vi "Property Read.vi"(4 "error in (no error)":errorcluster, 6 "Container State":T2, 7 "Display State In":T1={"Update"=FALSE, "Show advanced"=FALSE, "Fs (Hz)"=100000.0, "Show persist"=FALSE}) -> (0 "error out":errorcluster, 2 "Value":bool, 3 "Display State Out":T1={"Update"=FALSE, "Show advanced"=FALSE, "Fs (Hz)"=100000.0, "Show persist"=FALSE})   [LabVIEW 2015, in "Stimulus Channel (Full).xctl"]
uses:
  Stimulus Channel (Full).xctl
  <vilib>/_xctls/Container State.ctl
  State.ctl
  <vilib>/_xctls/XControlSupport.lvlib
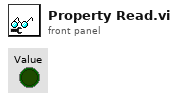
[diagram p1: front panel]
types:
  T1 = typedef "Stimulus Channel (Full).xctl/State.ctl" = cluster{"Update":bool, "Show advanced":bool, "Fs (Hz)":dbl, "Show persist":bool}
  T2 = typedef "XControlSupport.lvlib/Container State.ctl" = cluster{"Indicator?":bool, "Run Mode?":bool, " Refnum":refnum<vi>}
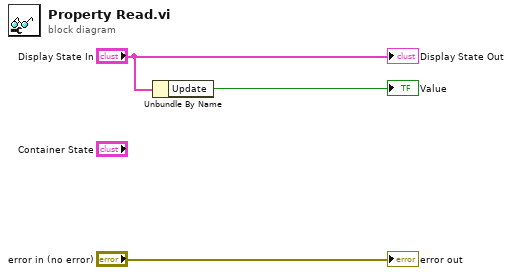
[diagram p0: block diagram]
diagram:
  n1 = Unbundle By Name("Display State In") -> ("Update"=→"Value":bool)
  "error out" <- "error in (no error)"
  "Display State Out" <- "Display State In"
